vi "IrIntializeDFScript.vi"(8 "error in (no error)":errorcluster) -> (0 "error out":errorcluster)   [LabVIEW 2017]
uses:
  <vilib>/addons/InsightCM/Devices/Shared/Common/DataFlow/controls/Type.ctl
  <vilib>/addons/InsightCM/Devices/Shared/Common/Trigger/Trigger.lvlib
  <vilib>/addons/InsightCM/Devices/Shared/Common/DataFlow/DataFlow.lvlib
  <vilib>/addons/InsightCM/Devices/Shared/Common/FileFlow/FileFlow.lvlib
  <vilib>/addons/InsightCM/Devices/Shared/Ir/IrAnalysis/IrAnalysis.lvlib
  <vilib>/addons/InsightCM/Devices/Shared/Common/TrendAlarm/TrendAlarm.lvlib
  <vilib>/addons/InsightCM/Devices/Shared/Ir/IrDataEventCreator/IrDataEventCreator.lvlib
  <vilib>/addons/InsightCM/Devices/Shared/Ir/IrTestPanel/IrTestPanel.lvlib
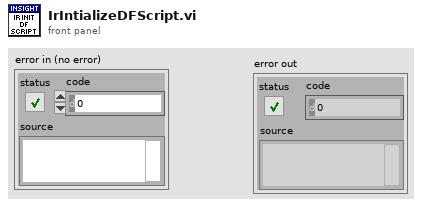
[diagram p1: front panel]
types:
  T1 = typedef "DataFlow.lvlib/Type.ctl" = enum16{"High Rate", "Low Rate", "Burst Mode"}
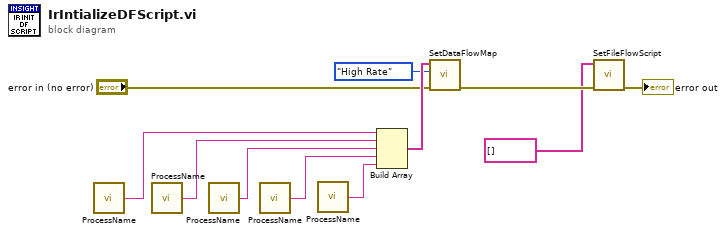
[diagram p0: block diagram]
diagram:
  n1 = call <vilib>:"ProcessName.vi"() -> ("process name"=w6:string)  [unwired: 5 in]
  n2 = call <vilib>:"ProcessName.vi"() -> ("process name"=w11:string)  [unwired: 5 in]
  n3 = call <vilib>:"ProcessName.vi"() -> ("process name"=w5:string)  [unwired: 5 in]
  n4 = call <vilib>:"ProcessName.vi"() -> ("process name"=w3:string)  [unwired: 5 in]
  n5 = call <vilib>:"ProcessName.vi"() -> ("process name"=w2:string)  [unwired: 5 in]
  n6 = Build Array(w6, w11, w5, w3, w2) -> (w10:string[])
  n7 = call <vilib>:"SetDataFlowMap.vi"("error in (no error)"="error in (no error)", "type"=Type."High Rate", "Dataflow script"=w10) -> ("error out"=w8:errorcluster)  [unwired: 8 in]
  n8 = call <vilib>:"SetFileFlowScript.vi"("error in (no error)"=w8, "Fileflow script"=string[] []) -> ("error out"=→"error out":errorcluster)  [unwired: 9 in]
